vi "getAllDescendants.vi"(11 "parentsIn":refnum<vi>[](array[refnum])) -> (1 "allNames":string[](array[string]), 2 "allDescendants":refnum<vi>[](array[refnum]), 3 "name-RefArray":T1(array[cluster]))   [LabVIEW 2021]
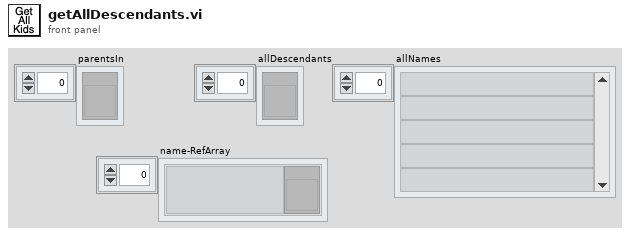
[diagram p1: front panel]
types:
  T1 = cluster{"Name":string, "Scene:Read Scene File":refnum<vi>}[]
  T2 = cluster{"Name":string, "Scene:Read Scene File":refnum<vi>}
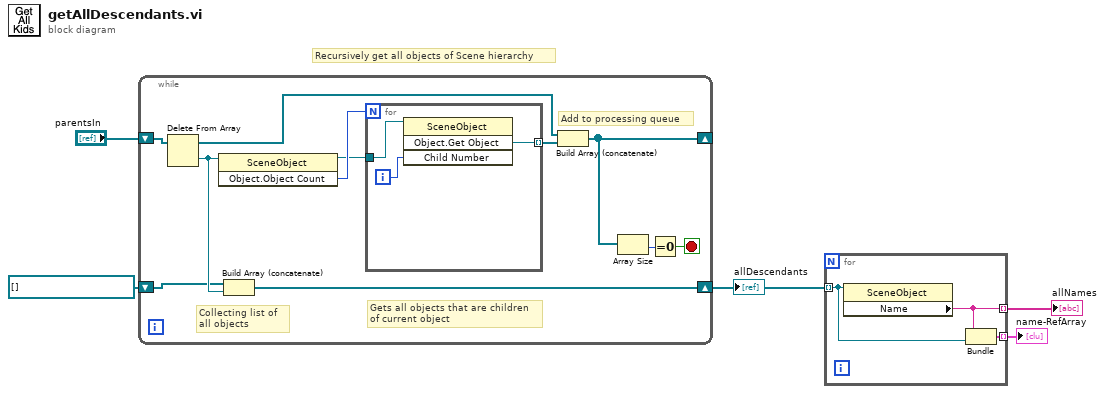
[diagram p0: block diagram]
diagram:
  # "Recursively get all objects of Scene hierarchy"
  n1 = while {
    shift-right: [w14] -> w3
    shift-left: refnum<vi>[] [] -> [w13]
    shift-right: [w8] -> _
    shift-left: "parentsIn" -> [w16]
    stop <- w6 stop-if-true
    # "Collecting list of \nall objects"
    # "Add to processing queue"
    # "Gets all objects that are children\nof current object"
    n2 = Delete From Array(array=w16) -> (deleted portion=w15:refnum<vi>, array with subset deleted=w9:refnum<vi>[])  [unwired: 2 in]
    n3 = invoke class="SceneObject" method="Object.Object Count"(reference=w15) -> (reference out=w11:refnum<vi>, "Child Count"=w12:i32)  [unwired: 2 in, 1 out]
    n4 = Build Array (concatenate)(w13, w15) -> (w14:refnum<vi>[])
    n5 = for {
      N: w12 -> [_]
      tunnel: w11 -> [w19]
      tunnel: [w17] -> w10 mode=indexing
      i -> [w18]
      n6 = invoke class="SceneObject" method="Object.Get Object"(reference=w19, "Child Number"=w18) -> ("Get Child"=w17:refnum<vi>)  [unwired: 2 in, 3 out]
    }
    n7 = Build Array (concatenate)(w9, w10) -> (w8:refnum<vi>[])
    n8 = Array Size(array=w8) -> (size(s)=w7:i32)
    n9 = Equal To 0?(x=w7) -> (x = 0?=w6:bool)
  }
  "allDescendants" <- w3
  n10 = for {
    tunnel: w3 -> [w21] mode=indexing
    tunnel: [w22] -> w2 mode=indexing
    tunnel: [w20] -> w1 mode=indexing
    n11 = property class="SceneObject"(reference=w21) -> ("Name"=w22:string)  [unwired: 1 in, 2 out]
    n12 = Bundle("Name"=w22, "Scene:Read Scene File"=w21) -> (w20:T2)  [unwired: 1 in]
  }
  "allNames" <- w2
  "name-RefArray" <- w1
